vi "niRFUtil FTW Generate RRC Response.vi"(0 "Center Frequency (0 Hz)":dbl format="%^.2e", 5 "Bandwidth (Hz)":dbl format="%^.2e", 7 "df (Hz)":dbl format="%^.2e", 9 "Minimum Selectivity (dB)":dbl=70.0 format="%.2f", 11 "Alpha":T3=0.22 format="%.3g") -> (4 "Filter Power Response":T1 {"y" min=0 max=127 format="%.2f"; "dx" format="%^.2e"; "x0" format="%^.2e"}, 6 "-ENBW (dB-Hz)":sgl format="%.2f")   [LabVIEW 2015, in "niRFUtil.lvlib"]
doc: "(c) Copyright 2006, National Instruments, Inc. This VI may not be duplicated, sold, or distributed without written consent from National Instruments."
uses:
  niRFUtil.lvlib
  Includes/niRFUtil INC RRC Filter Alpha.ctl
  Includes/niRFUtil INC Real Waveform.ctl
  Includes/niRFUtil INC Real Array.ctl
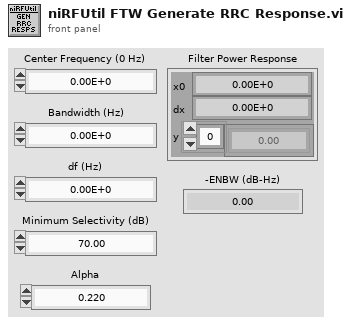
[diagram p1: front panel]
types:
  T1 = typedef "niRFUtil.lvlib/niRFUtil INC Real Waveform.ctl" = cluster{"x0":dbl, "dx":dbl, "y":T2}
  T2 = typedef "niRFUtil.lvlib/niRFUtil INC Real Array.ctl" = sgl[]
  T3 = typedef "niRFUtil.lvlib/niRFUtil INC RRC Filter Alpha.ctl" = dbl
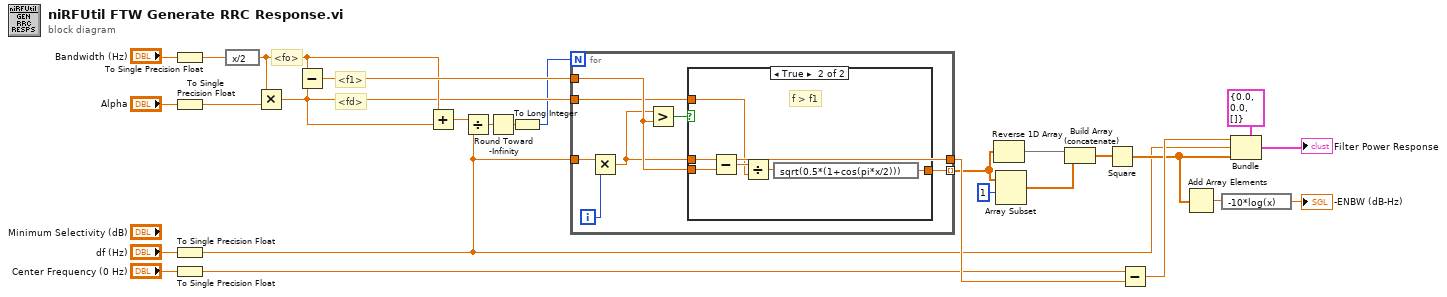
[diagram p0: block diagram]
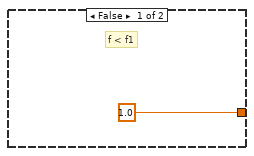
[diagram p2: hidden frame]
diagram:
  # "<f1>"
  # "<fd>"
  # "<fo>"
  n1 = To Single Precision Float(number="Bandwidth (Hz)") -> (single precision float=w14:sgl)
  n2 = To Single Precision Float(number="Alpha") -> (single precision float=w9:sgl)
  n3 = To Single Precision Float(number="df (Hz)") -> (single precision float=w5:sgl)
  n4 = To Single Precision Float(number="Center Frequency (0 Hz)") -> (single precision float=w11:sgl)
  n5 = expression code="x/2"(w14) -> (w21:sgl)
  n6 = Multiply(x=w21, y=w9) -> (x*y=w20:sgl)
  n7 = Subtract(x=w21, y=w20) -> (x-y=w24:sgl)
  n8 = Add(x=w21, y=w20) -> (x+y=w19:sgl)
  n9 = Divide(x=w19, y=w5) -> (x/y=w26:sgl)
  n10 = Round Toward -Infinity(1:w26) -> (0:w25:sgl)
  n11 = To Long Integer(number=w25) -> (32bit integer=w2:i32)
  n12 = for {
    N: w2 -> [_]
    tunnel: w24 -> [w33]
    tunnel: w20 -> [w32]
    tunnel: [w31] -> w3 mode=indexing
    tunnel: [w30] -> w18
    tunnel: w5 -> [w29]
    i -> [w28]
    n13 = Multiply(x=w29, y=w28) -> (x*y=w30:sgl)
    n14 = Greater?(x=w30, y=w33) -> (0:w34:bool)
    n15 = case shown="True" w34 {
      tunnel: w30 -> [_ w40]
      tunnel: w33 -> [_ w39]
      tunnel: w32 -> [_ w37]
      tunnel: [sgl 1.0 w36] -> w31
      frame False {
        # "f < f1"
      }
      frame True {
        # "f > f1"
        n16 = Subtract(x=w40, y=w39) -> (x-y=w38:sgl)
        n17 = Divide(x=w38, y=w37) -> (x/y=w41:sgl)
        n18 = expression code="sqrt(0.5*(1+cos(pi*x/2)))"(w41) -> (w36:sgl)
      }
    }
  }
  n19 = Reverse 1D Array(array=w3) -> (reversed array=w4:sgl[])
  n20 = Array Subset(array=w3, index=1) -> (w22:sgl[])  [unwired: 1 in]
  n21 = Build Array (concatenate)(w4, w22) -> (w1:sgl[])
  n22 = Square(x=w1) -> (x^2=w8:sgl[])
  n23 = Subtract(x=w11, y=w18) -> (x-y=w17:sgl)
  n24 = Add Array Elements(numeric array=w8) -> (sum=w7:sgl)
  n25 = expression code="-10*log(x)"(w7) -> (→"-ENBW (dB-Hz)":sgl)
  n26 = Bundle(cluster=T1 {"x0"=0.0, "dx"=0.0, "y"=[]} ("Filter"), "x0"=w17, "dx"=w5, "y"=w8) -> (→"Filter Power Response":T1)
